vi "Get Bmp File Header.vi"(8 "错误输入（无错误）":errorcluster, 11 "Bmp Data In":string) -> (0 "错误输出":errorcluster, 1 "Offset":i32, 2 "Bitmap Header":T1 {"bfOffBits" format="%.0x"; "bfSize" format="%.0x"; "bfType" format="%.0x"}, 3 "Bmp Data Out":string)   [LabVIEW 2012, in "Picture Box Tools.lvlib" / "BMP File.lvlib"]
uses:
  BMP File.lvlib
  Bmp File Header.ctl
panel:
  in  "BitmapHeader":T1 {"bfOffBits" format="%.0x"; "bfSize" format="%.0x"; "bfType" format="%.0x"}
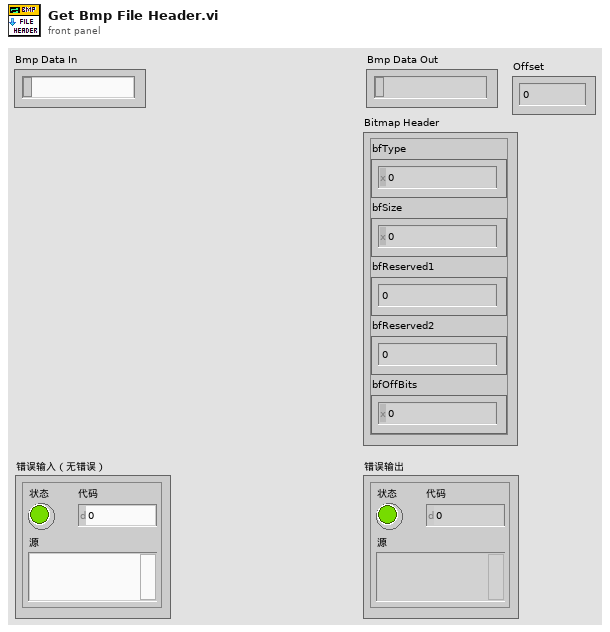
[diagram p1: front panel]
types:
  T1 = typedef "Picture Box Tools.lvlib/BMP File.lvlib/Bmp File Header.ctl" = cluster{"bfType":u16, "bfSize":u32, "bfReserved1":u16, "bfReserved2":u16, "bfOffBits":u32}
  T2 = enum16{"big-endian, network order", "native, host order", "little-endian"}
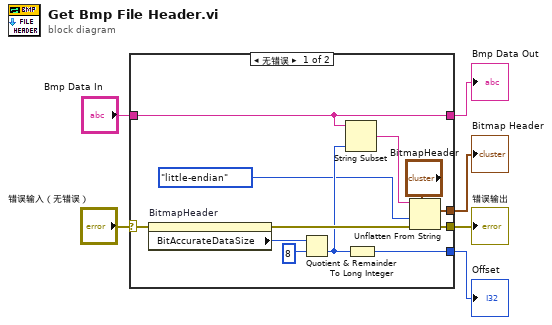
[diagram p0: block diagram]
diagram:
  n1 = case shown="无错误" "错误输入（无错误）" {
    selector: "错误输入（无错误）" -> [w14 w20]
    tunnel: "Bmp Data In" -> [w10 w19]
    tunnel: [w11 w20] -> w4
    tunnel: [w13 _] -> w3
    tunnel: [w10 w19] -> w2
    tunnel: [w7 _] -> w1
    frame No Error {
      n2 = property on="BitmapHeader" class="Clust (严格)"(error in=w14) -> (error out=w12:errorcluster, "BitAccurateDataSize"=w18:u32)  [unwired: 1 in, 1 out]
      n3 = Quotient & Remainder(x=w18, y=u32 8) -> (floor(x/y)=w9:u32)  [unwired: 1 out]
      n4 = String Subset(string=w10, length (rest)=w9) -> (substring=w15:string)  [unwired: 1 in]
      n5 = To Long Integer(number=w9) -> (32bit integer=w7:i32)
      n6 = Unflatten From String(type="BitmapHeader", binary string=w15, byte order (0:big-endian, network order)=T2."little-endian" ("字节顺序(0:big-endian, network order)"), error in (no error)=w12) -> (value=w13:T1, error out=w11:errorcluster)  [unwired: 1 in, 1 out]
    }
    frame Error {
    }
  }
  "错误输出" <- w4
  "Bitmap Header" <- w3
  "Bmp Data Out" <- w2
  "Offset" <- w1
